vi "MagBoard_Processor_n128.vi"() -> ()   [LabVIEW 2018]
uses:
  <vilib>/Math Plots/3D Math Plots/3D Surface/3D Surface XCtrl/3D Surface.xctl
  subVIs/calibration/FGVs/FGV States.ctl
  <vilib>/Utility/file.llb/Write Delimited Spreadsheet (DBL).vi
  <vilib>/Utility/file.llb/Read Delimited Spreadsheet (I64).vi
  <vilib>/Math Plots/3D Math Plots/3D Surface/3D Surface Datatype/Public/Plot Helper (Matrix).vi
  <vilib>/Math Plots/3D Math Plots/3D Surface/3D Surface Datatype/3D Surface Datatype.lvclass
panel:
  in  "Lookup_Indices":path=path "C:/Users/menprc/Documents/GitHub/MagLib/MagBoard_n64_UI/MagBoard_n64_UI_LabVIEW_Client/example_data/M064_008_up.dat"
  out "3D Surface":refnum<class "3D Plot Datatype.lvclass">[](xcontrol)
  out "Node XYZ List":dbl[][](array[numeric])
  out "dT":u32=4294745741
  in  "Calibration File":string="6x0-5mm"
  in  "Save Data":bool=TRUE
  in  "Export File (CSV)":path=path "C:/Users/menprc/Documents/GitHub/MagLib/MagBoard_n64_UI/MagBoard_n64_UI_LabVIEW_Client/example_data/M064_008.csv"
  in  "dT":u32=10
  out "Time":u32=4294745741
  in  "stop":bool
  in  "Data File":path=path "C:/Users/menprc/Documents/GitHub/MagLib/MagBoard_n64_UI/MagBoard_n64_UI_LabVIEW_Client/example_data/M064_008_up.dat"
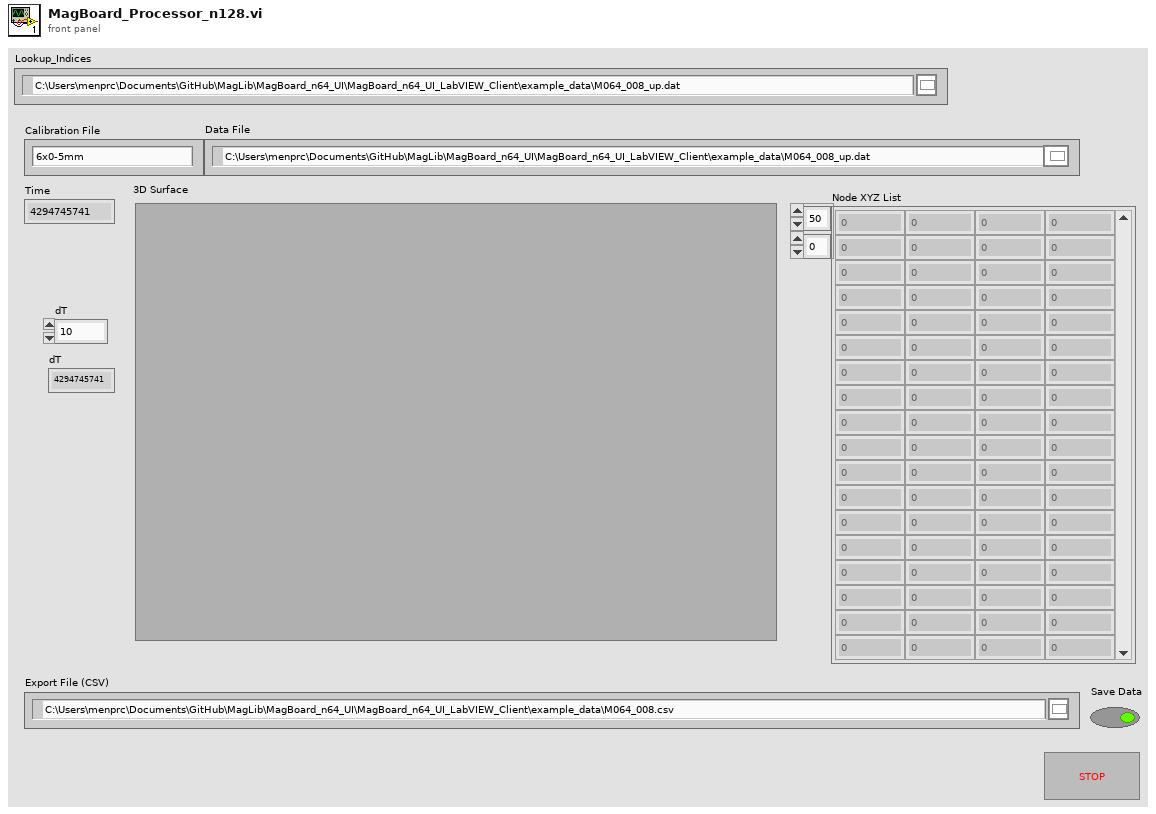
[diagram p1: front panel]
types:
  T1 = typedef "FGV States.ctl" = enum16{"Get", "Set", "Reset"}
  T2 = cluster{cluster{dbl[][], "Array":dbl[][]}, cluster{dbl[][], "Array":dbl[][]}, cluster{dbl[][], "Array":dbl[][]}, cluster{dbl[][], "Array":dbl[][]}}
  T3 = cluster{cluster{dbl[][], "Array":dbl[][]}, cluster{dbl[][], "Array":dbl[][]}, cluster{dbl[][], "Array":dbl[][]}, cluster{dbl[][], "Array":dbl[][]}}[]
  T4 = enum16{"big-endian, network order", "native, host order", "little-endian"}
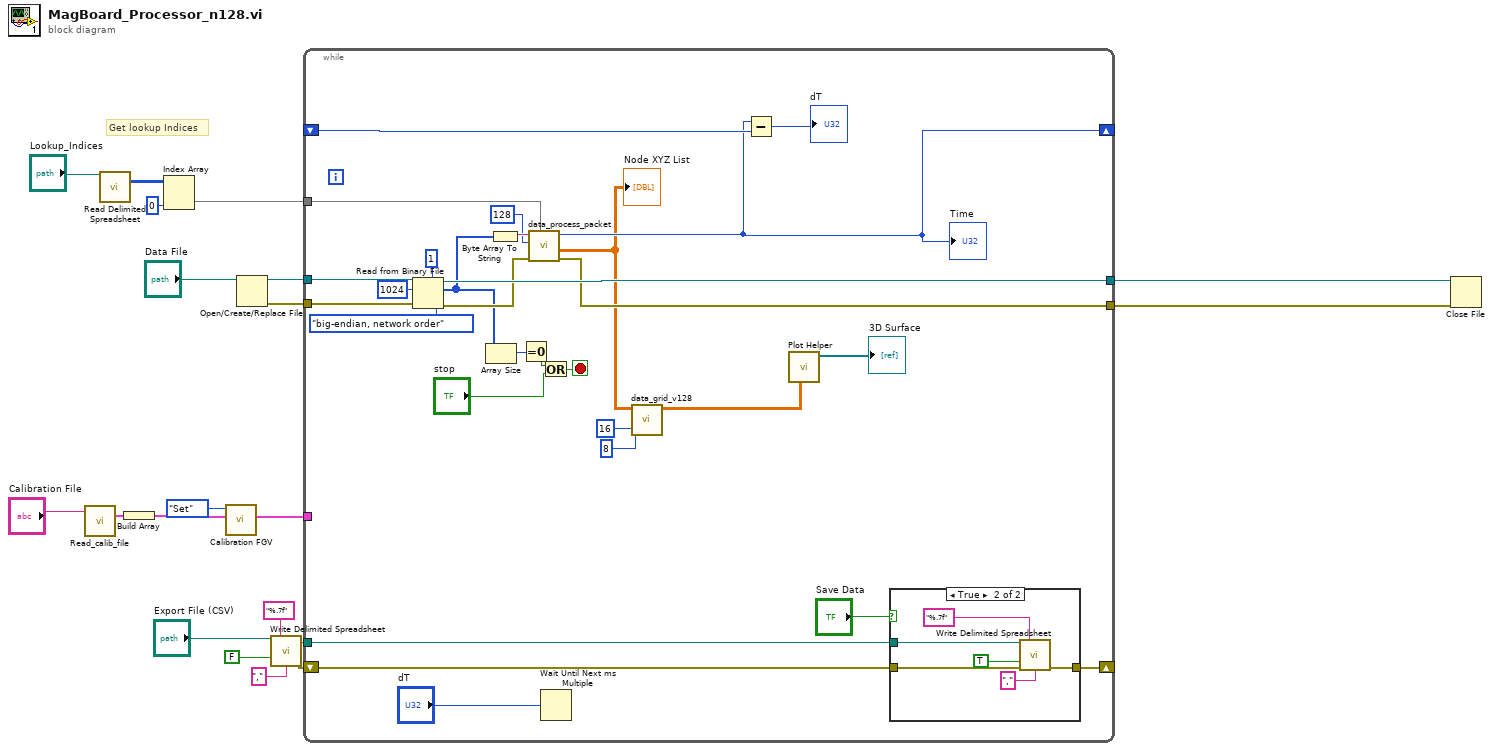
[diagram p0: block diagram]
diagram:
  # "Get lookup Indices"
  n1 = call "Read_calib_file.vi"("string"="Calibration File") -> ("output cluster"=w8:T2)  [unwired: 6 in, 4 out]
  n2 = call-poly <vilib>:"Read Delimited Spreadsheet.vi"("file path (dialog if empty)"="Lookup_Indices") -> ("all rows"=w3:i64[][])  [unwired: 9 in, 5 out]
  n3 = Build Array(w8) -> (w7:T3)
  n4 = Index Array(array=w3, index (col)=0 ("disabled index (col)")) -> (element=w1:i64[])  [unwired: 1 in]
  n5 = call "Calibration FGV.vi"("Calib in"=w7, "FGV States"=FGV_States."Set") -> ("Calib in 2"=w5:T3)  [unwired: 9 in]
  n6 = Open/Create/Replace File(file path (use dialog)="Data File") -> (refnum out=w19:refnum<file>, error out=w18:errorcluster)  [unwired: 5 in, 1 out]
  n7 = call-poly <vilib>:"Write Delimited Spreadsheet.vi"("file path (dialog if empty)"="Export File (CSV)", "format (%.3f)"="%.7f", "append to file? (new file:F)"=FALSE, "delimiter (\\t)"="," ("delimiter (\\t)")) -> ("new file path (Not A Path if cancelled)"=w12:path, "error out"=w10:errorcluster)  [unwired: 10 in]
  n8 = while {
    tunnel: w19 -> [w49]
    tunnel: w18 -> [w48]
    tunnel: [w46] -> w16
    tunnel: [w41] -> w17
    tunnel: w12 -> [w39]
    shift-right: [w37] -> _
    shift-left: w10 -> [w38]
    tunnel: w5 -> [_]
    shift-right: [w29] -> _
    shift-left: _ -> [w30]
    tunnel: w1 -> [w21]
    stop <- w32 stop-if-true
    n9 = Read from Binary File(5:u8 1 ("count (1)"), 8:w48, 9:T4."big-endian, network order" ("byte order (0:big-endian, network order)"), 10:1024 ("count (1)"), 11:w49) -> (0:w42:errorcluster, 2:w35:u8[], 3:w46:refnum<file>)  [unwired: 1 in, 1 out]
    n10 = Array Size(array=w35) -> (size(s)=w34:i32)
    n11 = Byte Array To String(unsigned byte array=w35) -> (string=w43:string)
    n12 = Equal To 0?(x=w34) -> (x = 0?=w33:bool)
    n13 = call "data_process_packet.vi"("Sensor Lookup Indices"=w21, "error in (no error)"=w42, "No. Sensors"=128 ("No. Nodes"), "Binary Input Data"=w43) -> ("error out"=w41:errorcluster, "Raw Sensors N x XYZ"=w25:dbl[][], "Time"=w29:u32)  [unwired: 3 in, 2 out]
    "Time" <- w29
    "Node XYZ List" <- w25
    n14 = Or(x=w33, y="stop") -> (x .or. y?=w32:bool)
    n15 = Wait Until Next ms Multiple(millisecond multiple="dT") -> ()  [unwired: 1 out]
    n16 = call "data_grid_v128.vi"("No. Columns"=8, "No. Rows"=16 ("Row Length"), "Sensor Data"=w25) -> ("Z (GRID)"=w23:dbl[][])  [unwired: 5 in, 3 out]
    n17 = Subtract(x=w29, y=w30) -> (x-y=→"dT":u32)
    n18 = call-poly <vilib>:"Plot Helper.vi"("z matrix"=w23) -> ("3D Plot lvclass Array out"=→"3D Surface":refnum<class "3D Plot Datatype.lvclass">[])  [unwired: 5 in, 5 out]
    n19 = case shown="True" "Save Data" {
      tunnel: w39 -> [_ w53]
      tunnel: w38 -> [w50 w52]
      tunnel: [w50 w51] -> w37
      frame False {
      }
      frame True {
        n20 = call-poly <vilib>:"Write Delimited Spreadsheet.vi"("file path (dialog if empty)"=w53, "format (%.3f)"="%.7f", "append to file? (new file:F)"=TRUE, "error in (no error)"=w52, "delimiter (\\t)"="," ("delimiter (\\t)")) -> ("error out"=w51:errorcluster)  [unwired: 9 in, 1 out]
      }
    }
  }
  n21 = Close File(refnum=w16, error in=w17) -> ()  [unwired: 2 out]
